vi "checksampleworking.vi"(1 "Array":bool[](array[boolean])) -> (9 "Boolean":bool)   [LabVIEW 2012]
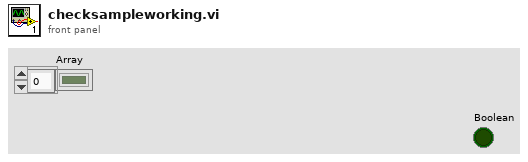
[diagram p1: front panel]
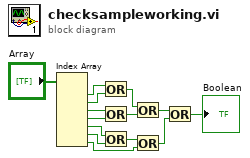
[diagram p0: block diagram]
diagram:
  n1 = Index Array(array="Array") -> (element #1=w7:bool, element #2=w6:bool, element #3=w5:bool, element #4=w4:bool, element #5=w3:bool, element #6=w2:bool, element #7=w1:bool)  [unwired: 7 in]
  n2 = Or(x=w7, y=w6) -> (x .or. y?=w14:bool)
  n3 = Or(x=w5, y=w4) -> (x .or. y?=w13:bool)
  n4 = Or(x=w3, y=w2) -> (x .or. y?=w12:bool)
  n5 = Or(x=w14, y=w13) -> (x .or. y?=w11:bool)
  n6 = Or(x=w12, y=w1) -> (x .or. y?=w10:bool)
  n7 = Or(x=w11, y=w10) -> (x .or. y?=→"Boolean":bool)
